vi "Display Console.vi"(8 "error in (no error)":errorcluster) -> (0 "error out":errorcluster)   [LabVIEW 2020]
doc: "Display Console Thread VI"
uses:
  Controls/Events_User.ctl
  Database/Controls/Account Database.ctl
  Controls/Data_Initialize.ctl
  <vilib>/Utility/error.llb/Error Cluster From Error Code.vi
  <vilib>/ErrorRing/Error Ring.xnode
  SubVIs/Message Queue/Message Queue.lvlib
  FGV/Controls/FGV_State.ctl
  Controls/Display Console.ctl
  Controls/Display Console Local Data.ctl
  SubVIs/Message Queue/Enqueue Message (Single).vi
  Controls/User Message.ctl
panel:
  out "Display Console":T1
  # "[Covers: UI1]"
  # "[CoversUI3B]"
  # "[CoversUI3C]"
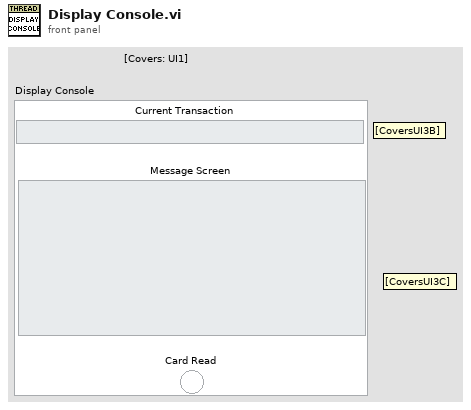
[diagram p1: front panel]
types:
  T1 = typedef "Display Console.ctl" = cluster{"Message Screen":string, "Card Read":bool, "Current Transaction":enum16{"", "Balance Inquiry", "Deposit", "Withdrawal", "Fast Cash $50", "New Transaction", "Terminate Session"}}
  T2 = enum32{"Invalid", "Standard", "Closed", "Hidden", "Minimized", "Maximized"}
  T3 = typedef "FGV_State.ctl" = enum16{"1 - OpenDatabase", "2 - Initialize Events", "3 - Initialize QMH", "4 - Close QMH", "5 - Close Events", "Read FGV", "Save Database", "Def"}
  T4 = typedef "FGV_Data.ctl" = cluster{"QMH":T5, "User Events":T6, "Database":T7[]}
  T5 = typedef "Message Queue.lvlib/All Message Queues.ctl" = cluster{"User Console":refnum<queue>, "Display Console":refnum<queue>, "Sensor Interface":refnum<queue>, "Process":refnum<queue>}
  T6 = typedef "Events_User.ctl" = cluster{"Stop User Console":refnum<user-event>, "Error User Console":refnum<user-event>, "Stop Sensor Interface ":refnum<user-event>, "Error Sensor Interface":refnum<user-event>}
  T7 = typedef "Account Database.ctl" = cluster{"Account Number":i32, "First Name":string, "Last Name":string, "Balance":dbl}
  T8 = typedef "User Message.ctl" = string[]
  T9 = typedef "Display Console Local Data.ctl" = cluster{"Initiliaze":T10, "Display Console":T1, "UserMessage":T8}
  T10 = typedef "Data_Initialize.ctl" = cluster{"Database":T7[], "User Events":T6}
  T11 = enum16{"Balance Inquiry", "Deposit", "Withdrawal", "Fast Cash $50", "New Transaction", "Terminate Session"}
  T12 = enum16{"", "Balance Inquiry", "Deposit", "Withdrawal", "Fast Cash $50", "New Transaction", "Terminate Session"}
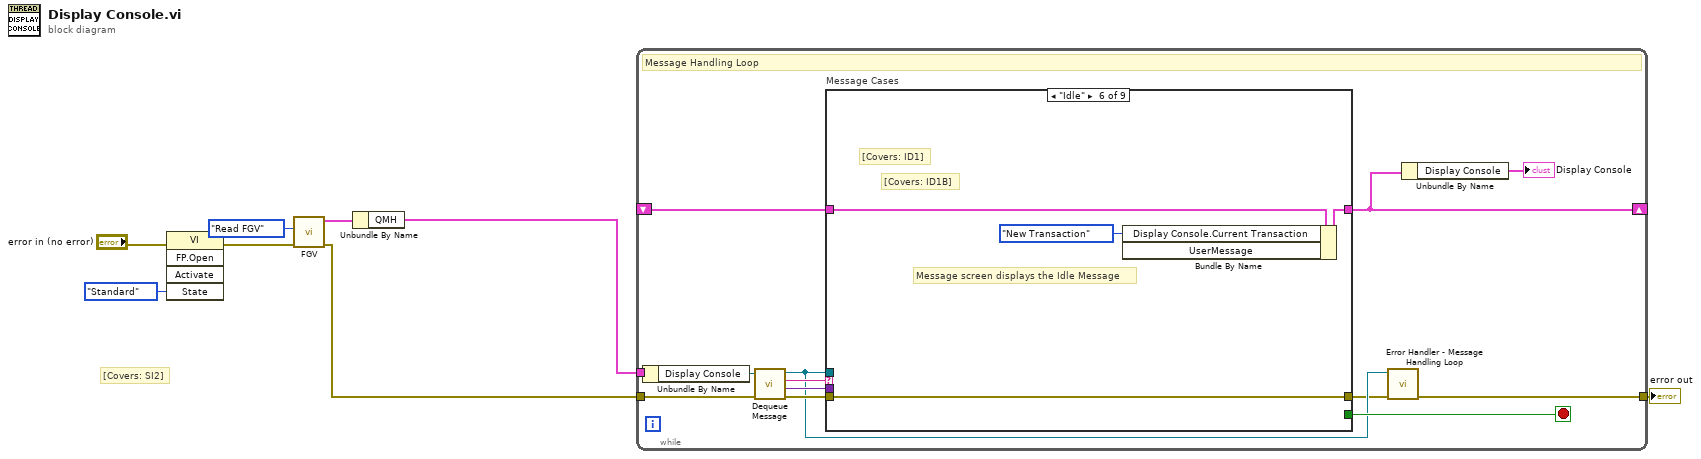
[diagram p0: block diagram]
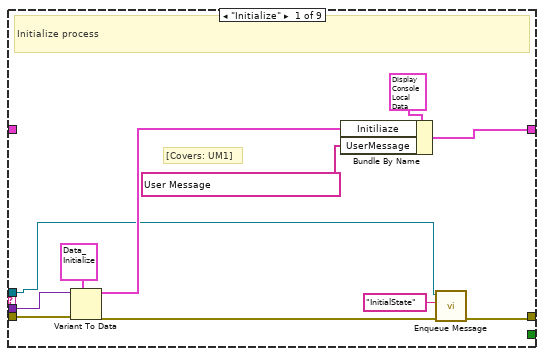
[diagram p2: hidden frame]
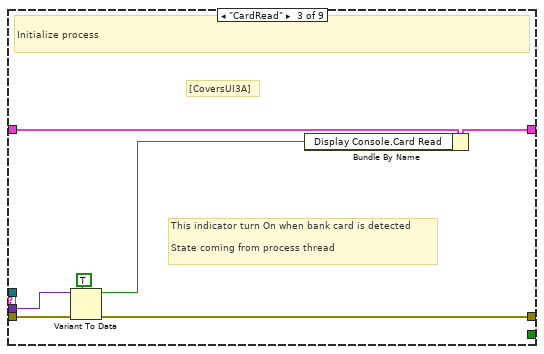
[diagram p4: hidden frame]
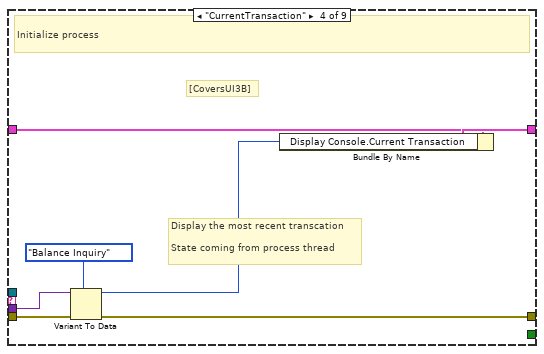
[diagram p5: hidden frame]
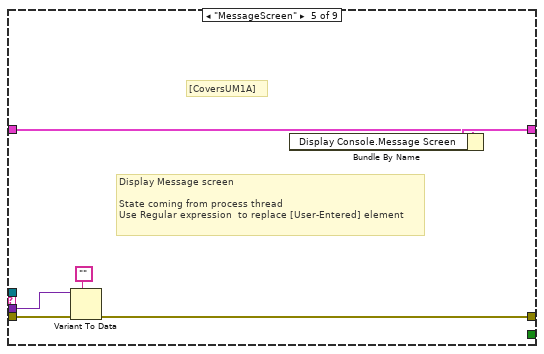
[diagram p6: hidden frame]
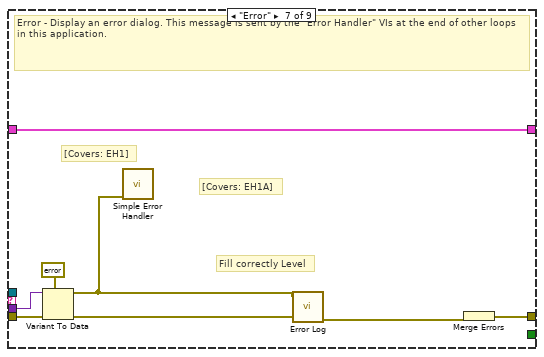
[diagram p7: hidden frame]
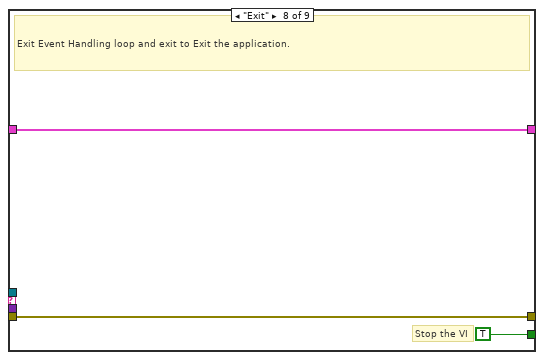
[diagram p8: hidden frame]
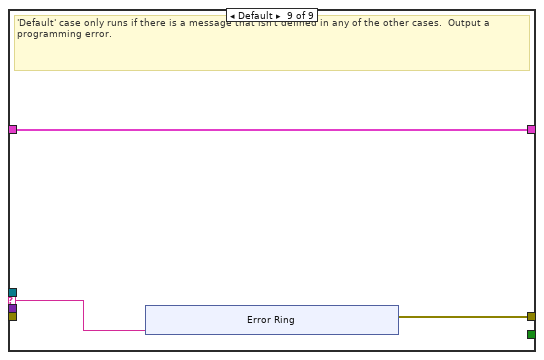
[diagram p9: hidden frame]
diagram:
  # "[Covers: SI2]"
  n1 = invoke class="VI" method="FP.Open"(error in="error in (no error)", "State"=T2."Standard") -> (error out=w4:errorcluster)  [unwired: 3 in, 4 out]
  n2 = call "FGV.vi"("error in (no error)"=w4, "FGV_State"=FGV_State."Read FGV") -> ("error out"=w1:errorcluster, "FGV 2"=w6:T4)  [unwired: 8 in]
  n3 = Unbundle By Name(w6) -> ("QMH"=w8:T5)
  n4 = while {
    tunnel: w8 -> [w12]
    shift-right: [w10] -> _
    shift-left: _ -> [w21]
    tunnel: w1 -> [w19]
    tunnel: [w14] -> w2
    stop <- w20 stop-if-true
    # "Message Handling Loop"
    n5 = Unbundle By Name(w12) -> ("Display Console"=w11:refnum<queue>)
    n6 = call "Dequeue Message.vi"("error in (no error)"=w19, "Message Queue"=w11) -> ("error out"=w18:errorcluster, "Message Data"=w16:variant, "Message"=w17:string, "dup Message Queue"=w15:refnum<queue>)  [unwired: 6 in]
    n7 = case "Message Cases" shown="\"Idle\"" w17 {
      selector: w17 -> [_ _ _ _ _ _ _ _ w70]
      tunnel: w15 -> [w24 _ _ _ _ _ _ _ _]
      tunnel: w18 -> [w31 w34 w40 w47 w53 w58 w66 w67 _]
      tunnel: [w23 w34 w38 w46 w49 w58 w62 w67 w71] -> w13
      tunnel: w21 -> [_ w33 w36 w44 w51 w57 w65 w68 w72]
      tunnel: [w32 w33 w41 w48 w54 w56 w65 w68 w72] -> w10
      tunnel: [_ _ _ _ _ _ _ TRUE _] -> w20
      tunnel: w16 -> [w28 _ w37 w45 w52 _ w64 _ _]
      frame "Initialize" {
        # "[Covers: UM1]"
        # "Initialize process"
        n8 = Variant To Data(error in=w31, type=T10 {"Database"=[], "User Events"={"Stop User Console"=refnum, "Error User Console"=refnum, "Stop Sensor Interface "=refnum, "Error Sensor Interface"=refnum}} ("Initiliaze"), Variant=w28) -> (data=w29:T10, error out=w25:errorcluster)
        n9 = Bundle By Name(cluster=T9 {"Initiliaze"={"Database"=[], "User Events"={"Stop User Console"=refnum, "Error User Console"=refnum, "Stop Sensor Interface "=refnum, "Error Sensor Interface"=refnum}}, "Display Console"={"Message Screen"="", "Card Read"=FALSE, "Current Transaction"=enum."Balance Inquiry"}, "UserMessage"=["Welcome to Acme Bank.\nPlease insert your card.", "Please enter your Account Number on the keypad.\nPress Enter (E) when done.\nAccount Number: [User-Entered]", "Welcome to Acme Bank\nFirst Name from DB, Last Name from DB\nPlease select a transaction by using the buttons.", "Account Information Incorrect\nPlease re-enter your Account Number.\nPress Enter (E) when done.\nAccount Number: [User-Entered]", "Your session has been terminated due to due to inactivity or menu selection.\nGoodbye!", "Please enter amount to deposit and press Enter (E) when done.\nDeposit Amount: $[User-Entered]", "Please enter amount to withdraw and press Enter (E) when done.\nWithdrawal Amount: $[User-Entered]", "", "Fast Cash $50 withdrawal processing", "Please remove cash from the ATM.", "Insufficient funds in account.\nPlease check your account balance and try again.", "Your Balance is:\n$ (Balance Amount from Database)"]} ("Local Data"), "Initiliaze"=w29, "UserMessage"=T8 ["Welcome to Acme Bank.\nPlease insert your card.", "Please enter your Account Number on the keypad.\nPress Enter (E) when done.\nAccount Number: [User-Entered]", "Welcome to Acme Bank\nFirst Name from DB, Last Name from DB\nPlease select a transaction by using the buttons.", "Account Information Incorrect\nPlease re-enter your Account Number.\nPress Enter (E) when done.\nAccount Number: [User-Entered]", "Your session has been terminated due to due to inactivity or menu selection.\nGoodbye!", "Please enter amount to deposit and press Enter (E) when done.\nDeposit Amount: $[User-Entered]", "Please enter amount to withdraw and press Enter (E) when done.\nWithdrawal Amount: $[User-Entered]", "", "Fast Cash $50 withdrawal processing", "Please remove cash from the ATM.", "Insufficient funds in account.\nPlease check your account balance and try again.", "Your Balance is:\n$ (Balance Amount from Database)"]) -> (w32:T9)
        n10 = call-poly "Enqueue Message.vi"("error in (no error)"=w25, "Message"="InitialState", "Message Queue"=w24) -> ("error out"=w23:errorcluster)  [unwired: 7 in, 1 out]
      }
      frame "InitialState" {
        # "Use reference to make card Read OFF\nCurrent Transaction OFF\nMessage Screnn Welcom message"
        # "[Covers: IS2]"
      }
      frame "CardRead" {
        # "[CoversUI3A]"
        # "This indicator turn On when bank card is detected \n\nState coming from process thread"
        # "Initialize process"
        n11 = Variant To Data(error in=w40, type=TRUE, Variant=w37) -> (data=w39:bool, error out=w38:errorcluster)
        n12 = Bundle By Name(cluster=w36, "Display Console.Card Read"=w39) -> (w41:T9)
      }
      frame "CurrentTransaction" {
        # "[CoversUI3B]"
        # "Display the most recent transcation \n\nState coming from process thread"
        # "Initialize process"
        n13 = Variant To Data(error in=w47, type=T11."Balance Inquiry" ("Display Console.Current Transaction"), Variant=w45) -> (data=w42:T11, error out=w46:errorcluster)
        n14 = Bundle By Name(cluster=w44, "Display Console.Current Transaction"=w42) -> (w48:T9)
      }
      frame "MessageScreen" {
        # "[CoversUM1A]"
        # "Display Message screen\n\nState coming from process thread\nUse Regular expression  to replace [User-Entered] element"
        n15 = Variant To Data(error in=w53, type="", Variant=w52) -> (error out=w49:errorcluster)  [unwired: 1 out]
        n16 = Bundle By Name(cluster=w51) -> (w54:T9)  [unwired: 1 in]
      }
      frame "Idle" {
        # "Message screen displays the Idle Message"
        # "[Covers: ID1B]"
        # "[Covers: ID1]"
        n17 = Bundle By Name(cluster=w57, "Display Console.Current Transaction"=T12."New Transaction") -> (w56:T9)  [unwired: 1 in]
      }
      frame "Error" {
        # "[Covers: EH1A]"
        # "[Covers: EH1]"
        # "Fill correctly Level"
        # "Error - Display an error dialog. This message is sent by the \"Error Handler\" VIs at the end of other loops in this application."
        n18 = Variant To Data(error in=w66, type=errorcluster {"status"=FALSE, "code"=0, "source"=""} ("error constant"), Variant=w64) -> (data=w59:errorcluster, error out=w61:errorcluster)
        n19 = call <vilib>:"Simple Error Handler.vi"("error in (no error)"=w59) -> ()  [unwired: 4 in, 5 out]
        n20 = call "Error Log.vi"("error in"=w61, "error happened"=w59) -> ("error out"=w60:errorcluster)  [unwired: 9 in]
        n21 = Merge Errors(w60) -> (w62:errorcluster)
      }
      frame "Exit" {
        # "Stop the VI"
        # "Exit Event Handling loop and exit to Exit the application."
      }
      frame Default {
        # "'Default' case only runs if there is a message that isn't defined in any of the other cases.  Output a programming error."
        n22 = xnode "Error Ring"("parameter 0"=w70) -> ("error out"=w71:errorcluster)
      }
    }
    n23 = call "Error Handler - Message Handling Loop.vi"("error in (no error)"=w13, "Message Queue"=w15) -> ("dup error in"=w14:errorcluster)  [unwired: 8 in, 1 out]
    n24 = Unbundle By Name(w10) -> ("Display Console"=→"Display Console":T1)
  }
  "error out" <- w2
